vi "Get Test Names and Results.vi"(8 "error in (no error)":errorcluster, 11 "Sequence Context In":T1) -> (0 "error out":errorcluster, 2 "Test Results":string[][](array[string]), 3 "Sequence Context Out":T1)   [LabVIEW 2010]
uses:
  <vilib>/addons/TestStand/_TSLegacy.llb/LabVIEW Test - Sequence Context.ctl
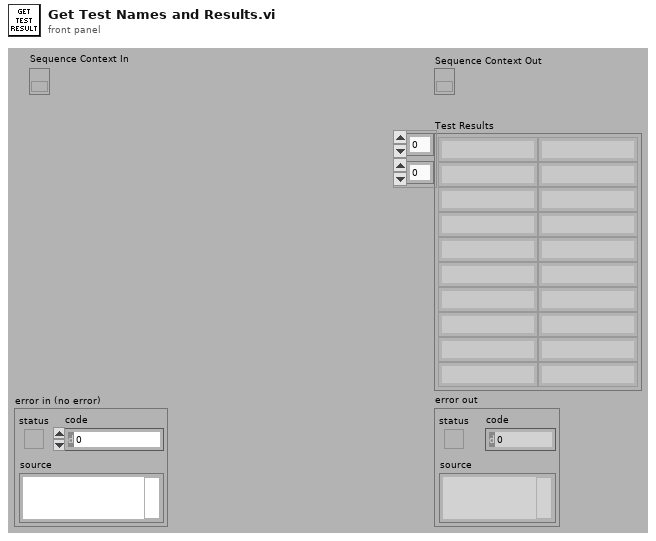
[diagram p1: front panel]
types:
  T1 = typedef "LabVIEW Test - Sequence Context.ctl" = refnum<k7>
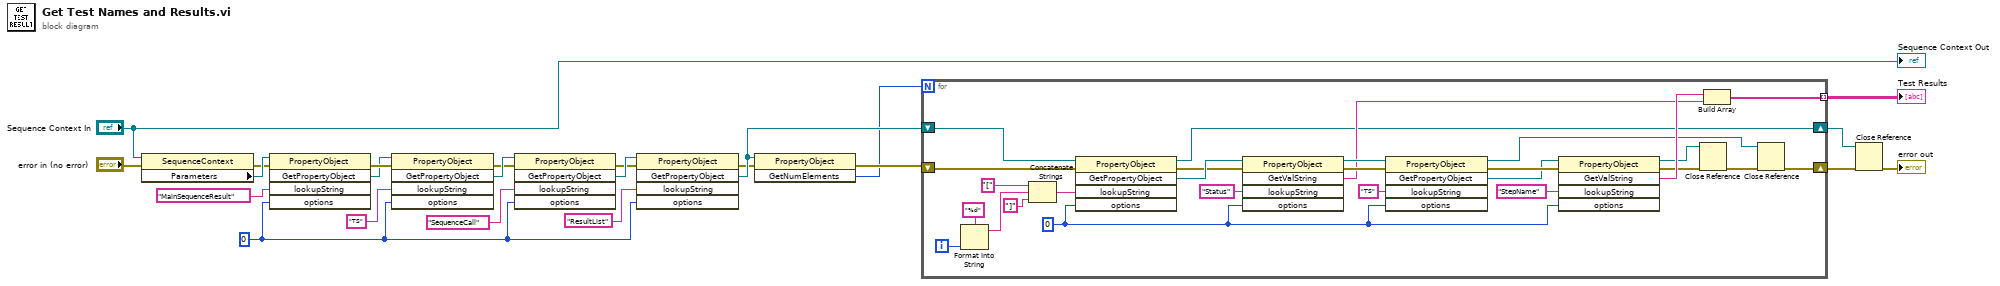
[diagram p0: block diagram]
diagram:
  w7 = 0 ("options")
  n1 = property class="SequenceContext"(reference="Sequence Context In", error in="error in (no error)") -> (error out=w18:errorcluster, "Parameters"=w19:refnum<k7>)  [unwired: 1 out]
  n2 = invoke class="PropertyObject" method="GetPropertyObject"(reference=w19, error in=w18, "lookupString"="MainSequenceResult", "options"=w7) -> (error out=w16:errorcluster, "GetPropertyObject"=w15:refnum<k7>)  [unwired: 1 in, 3 out]
  n3 = invoke class="PropertyObject" method="GetPropertyObject"(reference=w15, error in=w16, "lookupString"="TS", "options"=w7) -> (error out=w12:errorcluster, "GetPropertyObject"=w13:refnum<k7>)  [unwired: 1 in, 3 out]
  n4 = invoke class="PropertyObject" method="GetPropertyObject"(reference=w13, error in=w12, "lookupString"="SequenceCall", "options"=w7) -> (error out=w9:errorcluster, "GetPropertyObject"=w10:refnum<k7>)  [unwired: 1 in, 3 out]
  n5 = invoke class="PropertyObject" method="GetPropertyObject"(reference=w10, error in=w9, "lookupString"="ResultList", "options"=w7) -> (error out=w2:errorcluster, "GetPropertyObject"=w5:refnum<k7>)  [unwired: 1 in, 3 out]
  n6 = invoke class="PropertyObject" method="GetNumElements"(reference=w5, error in=w2) -> (error out=w4:errorcluster, "GetNumElements"=w1:i32)  [unwired: 1 in, 1 out]
  n7 = for {
    N: w1 -> [_]
    shift-right: [w26] -> w22
    shift-left: w4 -> [w40]
    tunnel: [w30] -> w23 mode=indexing
    shift-right: [w29] -> w20
    shift-left: w5 -> [w41]
    i -> [w38]
    w39 = 0 ("options")
    n8 = Format Into String(format string="%d", w38) -> (resulting string=w35:string)  [unwired: 2 in, 1 out]
    n9 = Concatenate Strings("[" ("lookupString"), w35, "]" ("string")) -> (w33:string)
    n10 = invoke class="PropertyObject" method="GetPropertyObject"(reference=w41, error in=w40, "lookupString"=w33, "options"=w39) -> (reference out=w29:refnum<k7>, error out=w45:errorcluster, "GetPropertyObject"=w47:refnum<k7>)  [unwired: 1 in, 2 out]
    n11 = invoke class="PropertyObject" method="GetValString"(reference=w47, error in=w45, "lookupString"="Status", "options"=w39) -> (reference out=w42:refnum<k7>, error out=w44:errorcluster, "GetValString"=w31:string)  [unwired: 1 in, 2 out]
    n12 = invoke class="PropertyObject" method="GetPropertyObject"(reference=w42, error in=w44, "lookupString"="TS", "options"=w39) -> (reference out=w24:refnum<k7>, error out=w50:errorcluster, "GetPropertyObject"=w48:refnum<k7>)  [unwired: 1 in, 2 out]
    n13 = invoke class="PropertyObject" method="GetValString"(reference=w48, error in=w50, "lookupString"="StepName", "options"=w39) -> (reference out=w25:refnum<k7>, error out=w27:errorcluster, "GetValString"=w32:string)  [unwired: 1 in, 2 out]
    n14 = Close Reference(reference=w25, error in (no error)=w27) -> (error out=w28:errorcluster)
    n15 = Build Array(w32, w31) -> (w30:string[])
    n16 = Close Reference(reference=w24, error in (no error)=w28) -> (error out=w26:errorcluster)
  }
  "Test Results" <- w23
  n17 = Close Reference(reference=w20, error in (no error)=w22) -> (error out=→"error out":errorcluster)
  "Sequence Context Out" <- "Sequence Context In"
